vi "UpdateMin&Max.vi"(9 "Numeric 24":dbl, 10 "Numeric 25":dbl, 11 "Cluster in":cluster{"SensorCluster":T1}) -> (3 "Cluster out":cluster{"SensorCluster":T1})   [LabVIEW 2018]
uses:
  Type_Def/Type_Def ClusterSensor.ctl
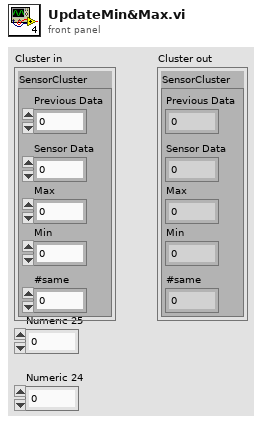
[diagram p1: front panel]
types:
  T1 = typedef "Type_Def ClusterSensor.ctl" = cluster{"Sensor Data":dbl, "Max":dbl, "Min":dbl, "Previous Data":dbl, "#same":dbl}
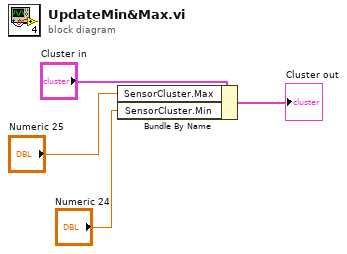
[diagram p0: block diagram]
diagram:
  n1 = Bundle By Name(cluster="Cluster in", "SensorCluster.Max"="Numeric 25", "SensorCluster.Min"="Numeric 24") -> (→"Cluster out":cluster{"SensorCluster":T1})
